vi "ADC_downsampling.vi"(1 "downsampling":u64, 2 "data in":dbl[][](array[numeric])) -> (0 "data out":dbl[][](array[numeric]))   [LabVIEW 2013]
uses:
  <vilib>/Analysis/baseanly.llb/Mean (DBL).vi
  <vilib>/Analysis/NI_AALBase.lvlib
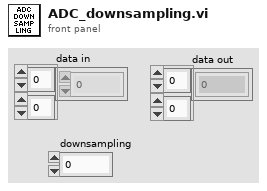
[diagram p1: front panel]
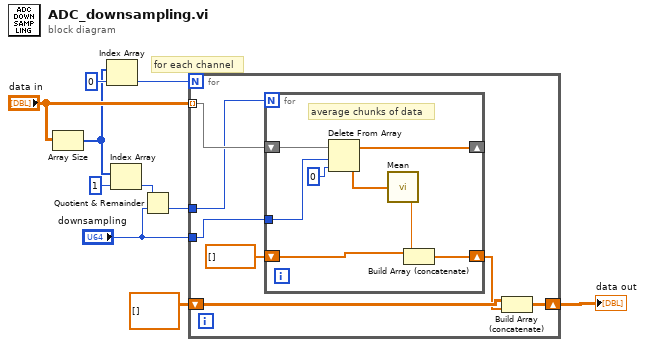
[diagram p0: block diagram]
diagram:
  # "for each channel"
  n1 = Array Size(array="data in") -> (size(s)=w4:i32[])
  n2 = Index Array(array=w4, index=0) -> (element=w6:i32)
  n3 = Index Array(array=w4, index=1) -> (element=w3:i32)
  n4 = Quotient & Remainder(x=w3, y="downsampling") -> (floor(x/y)=w1:u64)  [unwired: 1 out]
  n5 = for {
    N: w6 -> [_]
    tunnel: "data in" -> [w17] mode=indexing
    shift-right: [w15] -> w10
    shift-left: dbl[][] [] -> [w16]
    tunnel: "downsampling" -> [w13]
    tunnel: w1 -> [w12]
    n6 = for {
      N: w12 -> [_]
      shift-right: [w24] -> _
      shift-left: w17 -> [w25]
      shift-right: [w20] -> w14
      shift-left: dbl[] [] -> [w21]
      tunnel: w13 -> [w18]
      # "average chunks of data"
      n7 = Delete From Array(array=w25, length=w18, index=0) -> (deleted portion=w22:dbl[], array with subset deleted=w24:dbl[])
      n8 = call-poly <vilib>:"Mean.vi"("X"=w22) -> ("mean"=w19:dbl)  [unwired: 1 out]
      n9 = Build Array (concatenate)(w21, w19) -> (w20:dbl[])
    }
    n10 = Build Array (concatenate)(w16, w14) -> (w15:dbl[][])
  }
  "data out" <- w10
